vi "Initialize Sim youBot Gripper Motor.vi"(8 "error in (no error)":errorcluster, 11 "device ID":T1) -> (0 "error out":errorcluster, 3 "simulated KUKA youBot gripper motor out":refnum<class "NI_Robotics_KUKA youBot Gripper Motor_Sim.lvclass">)   [LabVIEW 2017, in "NI_Robotics_KUKA youBot Host.lvlib" / "NI_Robotics_KUKA youBot Gripper Motor_Sim.lvclass"]
uses:
  <vilib>/robotics/KUKA youBot/Motor/Gripper Motor Sim/NI_Robotics_KUKA youBot Gripper Motor_Sim.lvclass
  <vilib>/robotics/Simulator/Engine/ctl/DeviceID.ctl
  <vilib>/robotics/KUKA youBot/Motor/Gripper Motor Sim/NI_Robotics_KUKA youBot Gripper Motor_Sim.lvclass/NI_Robotics_KUKA youBot Gripper Motor_Sim.ctl
  <vilib>/robotics/Simulator/NI_Robotics_Simulator.lvlib
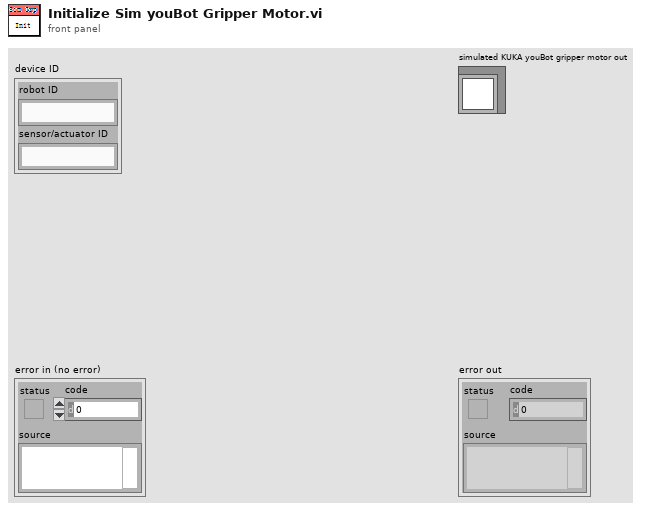
[diagram p1: front panel]
types:
  T1 = typedef "NI_Robotics_Simulator.lvlib/DeviceID.ctl" = cluster{"robot ID":string, "sensor/actuator ID":string}
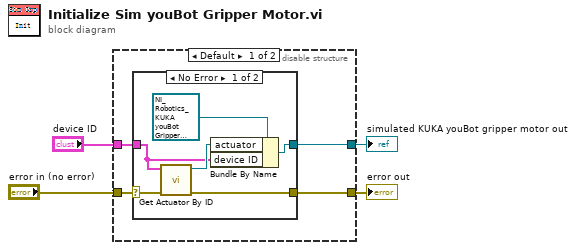
[diagram p0: block diagram]
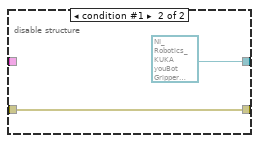
[diagram p3: hidden frame]
diagram:
  n1 = disable-structure shown="Default" {
    disable-tunnel: "error in (no error)" -> [w8 w17]
    disable-tunnel: [w7 w17] -> w2
    disable-tunnel: [w5 refnum<class "NI_Robotics_KUKA youBot Gripper Motor_Sim.lvclass"> refnum ("NI_Robotics_KUKA youBot Host.lvlib:NI_Robotics_KUKA youBot Gripper Motor_Sim.lvclass")] -> w1
    disable-tunnel: "device ID" -> [w6 _]
    frame condition #0 (active) {
      n2 = case shown="No Error" w8 {
        selector: w8 -> [w14 w15]
        tunnel: [w13 w15] -> w7
        tunnel: w6 -> [w9 _]
        tunnel: [w11 _] -> w5
        frame No Error {
          n3 = call <vilib>:"Get Actuator By ID.vi"("error in (no error)"=w14, "device ID"=w9) -> ("error out"=w13:errorcluster, "actuator class"=w12:refnum<class "ODESimulator_Motor.lvclass">)  [unwired: 8 in]
          n4 = Bundle By Name(cluster=refnum<class "NI_Robotics_KUKA youBot Gripper Motor_Sim.lvclass"> refnum ("NI_Robotics_KUKA youBot Host.lvlib:NI_Robotics_KUKA youBot Gripper Motor_Sim.lvclass"), "actuator"=w12, "device ID"=w9) -> (w11:refnum<class "NI_Robotics_KUKA youBot Gripper Motor_Sim.lvclass">)
        }
        frame Error {
        }
      }
    }
    frame condition #1 {
    }
  }
  "error out" <- w2
  "simulated KUKA youBot gripper motor out" <- w1
